vi "solar_voy_def Resolve Path.vi"(7 "Create Folder? (T)":bool=TRUE, 8 "error in (no error)":errorcluster, 9 "TARGET":string, 10 "PATH (..=Root)":T1, 11 "COSMOS_ROOT":path) -> (0 "error out":errorcluster, 3 "Resolved Path":path)   [LabVIEW 2018]
doc: "This resolves a COSMOS directory path."
uses:
  solar_voy_def_ctl PATH.ctl
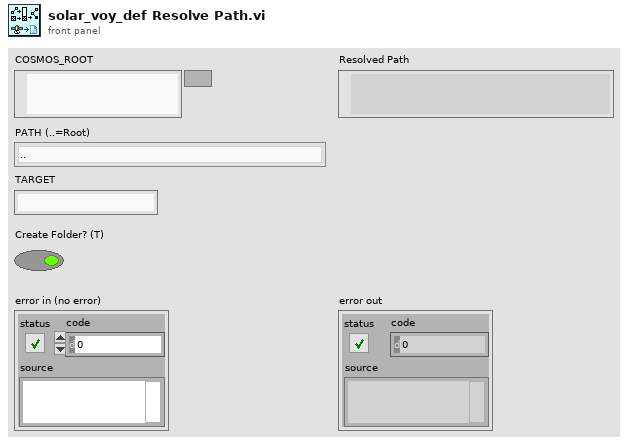
[diagram p1: front panel]
types:
  T1 = typedef "solar_voy_def_ctl PATH.ctl" = enum8{"..", "config", "config/data", "config/system", "config/targets", "config/targets/TARGET", "config/targets/TARGET/cmd_tlm", "config/targets/TARGET/lib", "config/targets/TARGET/screens", "config/tools", "config/tools/cmd_tlm_server", "config/tools/data_viewer", "config/tools/handbook_creator", "config/tools/launcher", "config/tools/limits_monitor", "config/tools/opengl_builder", "config/tools/script_runner", "config/tools/table_manager", "config/tools/test_runner", "config/tools/tlm_extractor", "config/tools/tlm_grapher", "config/tools/tlm_viewer", "lib", "outputs", "outputs/handbooks", "outputs/logs", "outputs/saved_config", "outputs/tables", "outputs/tmp", "procedures", "tools", "Launcher.bat", "config/system/system.txt", "config/targets/TARGET/cmd_tlm/TARGET_cmd.txt", "config/targets/TARGET/cmd_tlm/TARGET_tlm.txt", "config/targets/TARGET/cmd_tlm_server.txt", "config/targets/TARGET/target.txt", "config/tools/cmd_tlm_server/cmd_tlm_server.txt", "config/tools/data_viewer/data_viewer.txt", "config/tools/handbook_creator/handbook_creator.txt", "config/tools/launcher/launcher.txt", "config/tools/limits_monitor/limits_monitor.txt", "config/tools/opengl_builder/opengl_builder.txt", "config/tools/script_runner/script_runner.txt", "config/tools/table_manager/table_manager.txt", "config/tools/test_runner/test_runner.txt", "config/tools/tlm_extractor/tlm_extractor.txt", "config/tools/tlm_grapher/tlm_grapher.txt", "config/tools/tlm_viewer/tlm_viewer.txt"}
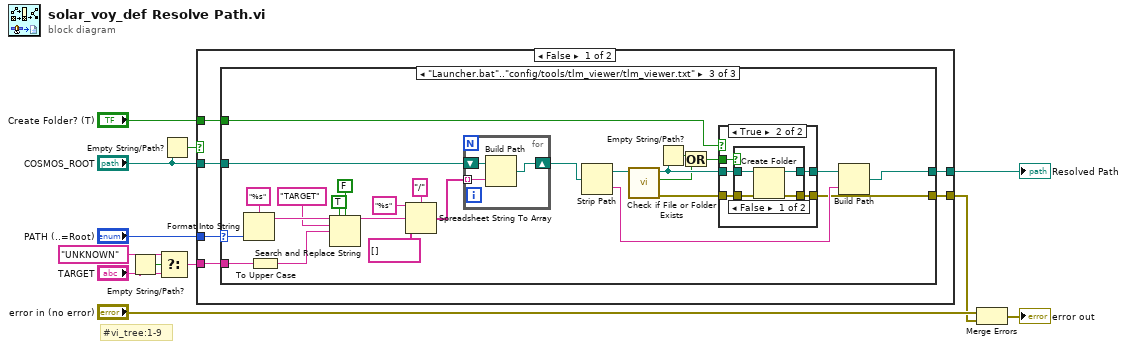
[diagram p0: block diagram]
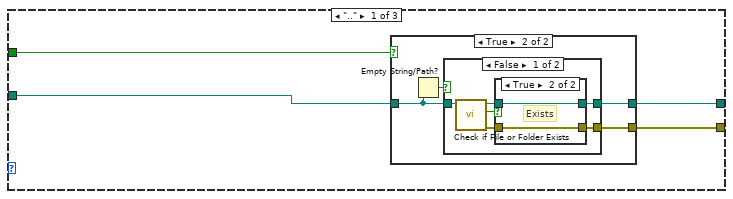
[diagram p2: hidden frame]
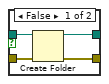
[diagram p4: hidden frame]
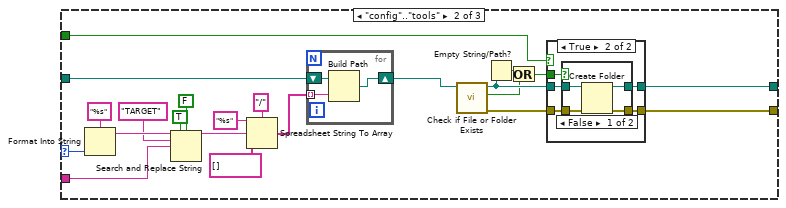
[diagram p6: hidden frame]
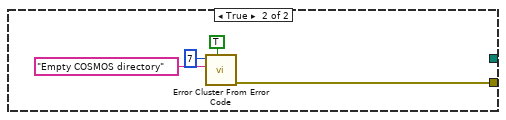
[diagram p11: hidden frame]
diagram:
  # "#vi_tree:1-9"
  n1 = Empty String/Path?(string/path="TARGET") -> (empty?=w6:bool)
  n2 = Select(t="UNKNOWN", s=w6, f="TARGET") -> (s? t:f=w4:string)
  n3 = Empty String/Path?(string/path="COSMOS_ROOT") -> (empty?=w1:bool)
  n4 = case shown="False" w1 {
    tunnel: "PATH (..=Root)" -> [w18 _]
    tunnel: [w17 _] -> w11
    tunnel: "COSMOS_ROOT" -> [w16 _]
    tunnel: "Create Folder? (T)" -> [w15 _]
    tunnel: [w14 w124] -> w7
    tunnel: w4 -> [w13 _]
    frame False {
      n5 = case shown="\"Launcher.bat\"..\"config/tools/tlm_viewer/tlm_viewer.txt\"" w18 {
        selector: w18 -> [_ w62 w104]
        tunnel: [w19 w49 w93] -> w17
        tunnel: w16 -> [w22 w57 w91]
        tunnel: w15 -> [w21 w41 w80]
        tunnel: w13 -> [_ w53 w96]
        tunnel: [w20 w50 w82] -> w14
        frame ".." {
          n6 = case shown="True" w21 {
            tunnel: w22 -> [w23 w25]
            tunnel: [_ w27] -> w20
            tunnel: [w23 w26] -> w19
            frame False {
            }
            frame True {
              n7 = Empty String/Path?(string/path=w25) -> (empty?=w24:bool)
              n8 = case shown="False" w24 {
                tunnel: w25 -> [w33 w40]
                tunnel: [w30 _] -> w27
                tunnel: [w29 w40] -> w26
                frame False {
                  n9 = call <vilib>:"Check if File or Folder Exists.vi"("path"=w33) -> ("error out"=w31:errorcluster, "file or folder exists?"=w28:bool, "dup path"=w32:path)  [unwired: 8 in]
                  n10 = case shown="True" w28 {
                    tunnel: w32 -> [w37 w38]
                    tunnel: w31 -> [w36 w39]
                    tunnel: [w35 w39] -> w30
                    tunnel: [w34 w38] -> w29
                    frame False {
                      n11 = Create Folder(path (use dialog)=w37, error in=w36) -> (created path=w34:path, error out=w35:errorcluster)  [unwired: 1 in, 1 out]
                    }
                    frame True {
                      # "Exists"
                    }
                  }
                }
                frame True {
                }
              }
            }
          }
        }
        frame "config".."tools" {
          n12 = Format Into String(format string="%s", w62) -> (resulting string=w56:string)  [unwired: 2 in, 1 out]
          n13 = Search and Replace String(replace all?=TRUE ("replace all? (F)"), case sensitive?=FALSE ("ignore case? (F)"), input string=w56, search string="TARGET", replace string=w53) -> (result string=w55:string)  [unwired: 3 in, 3 out]
          n14 = Spreadsheet String To Array(delimiter (Tab)="/", format string="%s", spreadsheet string=w55, array type (2D Dbl)=string[] []) -> (array=w47:string[])
          n15 = for {
            shift-right: [w77] -> w48
            shift-left: w57 -> [w78]
            tunnel: w47 -> [w76] mode=indexing
            n16 = Build Path(base path=w78, name or relative path=w76) -> (appended path=w77:path)
          }
          n17 = call <vilib>:"Check if File or Folder Exists.vi"("path"=w48) -> ("error out"=w46:errorcluster, "file or folder exists?"=w43:bool, "dup path"=w45:path)  [unwired: 8 in]
          n18 = Empty String/Path?(string/path=w45) -> (empty?=w44:bool)
          n19 = Or(x=w44, y=w43) -> (x .or. y?=w42:bool)
          n20 = case shown="True" w41 {
            tunnel: [w63 w69] -> w50
            tunnel: [w64 w68] -> w49
            tunnel: w46 -> [w63 w67]
            tunnel: w45 -> [w64 w66]
            tunnel: w42 -> [_ w65]
            frame False {
            }
            frame True {
              n21 = case shown="False" w65 {
                tunnel: w66 -> [w73 w74]
                tunnel: w67 -> [w72 w75]
                tunnel: [w71 w75] -> w69
                tunnel: [w70 w74] -> w68
                frame False {
                  n22 = Create Folder(path (use dialog)=w73, error in=w72) -> (created path=w70:path, error out=w71:errorcluster)  [unwired: 1 in, 1 out]
                }
                frame True {
                  # "Exists"
                }
              }
            }
          }
        }
        frame "Launcher.bat".."config/tools/tlm_viewer/tlm_viewer.txt" {
          n23 = Format Into String(format string="%s", w104) -> (resulting string=w99:string)  [unwired: 2 in, 1 out]
          n24 = To Upper Case(1:w96) -> (0:w79:string)
          n25 = Search and Replace String(replace all?=TRUE ("replace all? (F)"), case sensitive?=FALSE ("ignore case? (F)"), input string=w99, search string="TARGET", replace string=w79) -> (result string=w98:string)  [unwired: 3 in, 3 out]
          n26 = Spreadsheet String To Array(delimiter (Tab)="/", format string="%s", spreadsheet string=w98, array type (2D Dbl)=string[] []) -> (array=w89:string[])
          n27 = for {
            shift-right: [w119] -> w90
            shift-left: w91 -> [w120]
            tunnel: w89 -> [w118] mode=indexing
            n28 = Build Path(base path=w120, name or relative path=w118) -> (appended path=w119:path)
          }
          n29 = Strip Path(path=w90) -> (stripped path=w83:path, name=w92:string)
          n30 = call <vilib>:"Check if File or Folder Exists.vi"("path"=w83) -> ("error out"=w88:errorcluster, "file or folder exists?"=w85:bool, "dup path"=w87:path)  [unwired: 8 in]
          n31 = Empty String/Path?(string/path=w87) -> (empty?=w86:bool)
          n32 = Or(x=w86, y=w85) -> (x .or. y?=w84:bool)
          n33 = case shown="True" w80 {
            tunnel: [w105 w111] -> w82
            tunnel: [w106 w110] -> w81
            tunnel: w88 -> [w105 w109]
            tunnel: w87 -> [w106 w108]
            tunnel: w84 -> [_ w107]
            frame False {
            }
            frame True {
              n34 = case shown="False" w107 {
                tunnel: w108 -> [w115 w116]
                tunnel: w109 -> [w114 w117]
                tunnel: [w113 w117] -> w111
                tunnel: [w112 w116] -> w110
                frame False {
                  n35 = Create Folder(path (use dialog)=w115, error in=w114) -> (created path=w112:path, error out=w113:errorcluster)  [unwired: 1 in, 1 out]
                }
                frame True {
                  # "Exists"
                }
              }
            }
          }
          n36 = Build Path(base path=w81, name or relative path=w92) -> (appended path=w93:path)
        }
      }
    }
    frame True {
      n37 = call <vilib>:"Error Cluster From Error Code.vi"("show call chain? (False)"=TRUE, "error message (\"\")"="Empty COSMOS directory" ("error message (\"\")"), "error code (0)"=7) -> ("error out"=w124:errorcluster)  [unwired: 6 in]
    }
  }
  "Resolved Path" <- w11
  n38 = Merge Errors("error in (no error)", w7) -> (→"error out":errorcluster)
